vi "SEQ Monitoring Global Variables.vi"() -> ()   [LabVIEW 2014]
uses:
  SeqLoop/Classes/STEP/STEP.lvclass
  SeqLoop/TypeDefs/Sequence.ctl
  SeqLoop/TypeDefs/LogicParsedExpression.ctl
  SeqLoop/SeqLoop.lvlib
panel:
  in  "Current Sequence":T1
  in  "Current STEP":refnum<class "STEP.lvclass">
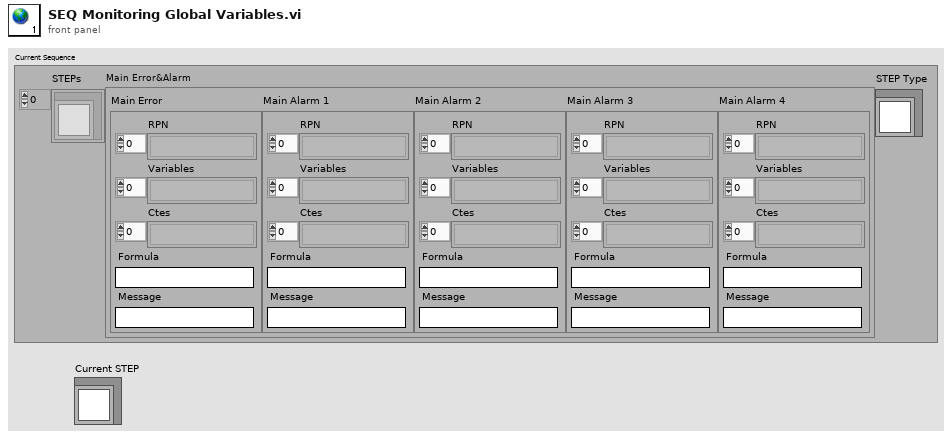
[diagram p1: front panel]
types:
  T1 = typedef "SeqLoop.lvlib/Sequence.ctl" = cluster{"STEPs":refnum<class "STEP.lvclass">[], "Main Error&Alarm":cluster{"Main Error":T2, "Main Alarm 1":T2, "Main Alarm 2":T2, "Main Alarm 3":T2, "Main Alarm 4":T2}, "STEP Type":refnum<class "STEP.lvclass">}
  T2 = typedef "SeqLoop.lvlib/LogicParsedExpression.ctl" = cluster{"RPN ":string[], "Variables":string[], "Ctes":string[], "Formula":string, "Message":string}
diagram:
